vi "Configure.vi"(8 "error in (no error)":errorcluster, 11 "Piezo in":refnum<class "Piezo.lvclass">) -> (0 "error out":errorcluster, 2 "cancelled?":bool, 3 "Piezo out":refnum<class "Piezo.lvclass">)   [LabVIEW 2012, in "Piezo.lvclass"]
doc: "The configure method configures the details for the RabbitMQ connection, the observers and the mapping script.\n\nIn the derived class, make a call to the parent for setting these parameters."
uses:
  Piezo.lvclass
  <vilib>/Utility/miscctls.llb/LVPointTypeDef.ctl
  Piezo.lvclass/Piezo.ctl
  <vilib>/Distrio/Murmex/Murmex/Murmex.lvclass
panel:
  in  "button:call parent":bool
  in  "button:ok":bool
  in  "button:cancel":bool
  in  "Tab Control":enum32{"Task"}(tab)
  in  "Min position":dbl[unit]
  in  "Max position":dbl[unit]
  in  "Reporting folder":path
  in  "Micron to voltage\nconversion factor":dbl[unit]
  in  "Min V":dbl
  in  "Max V":dbl
  in  "Analog output":tag
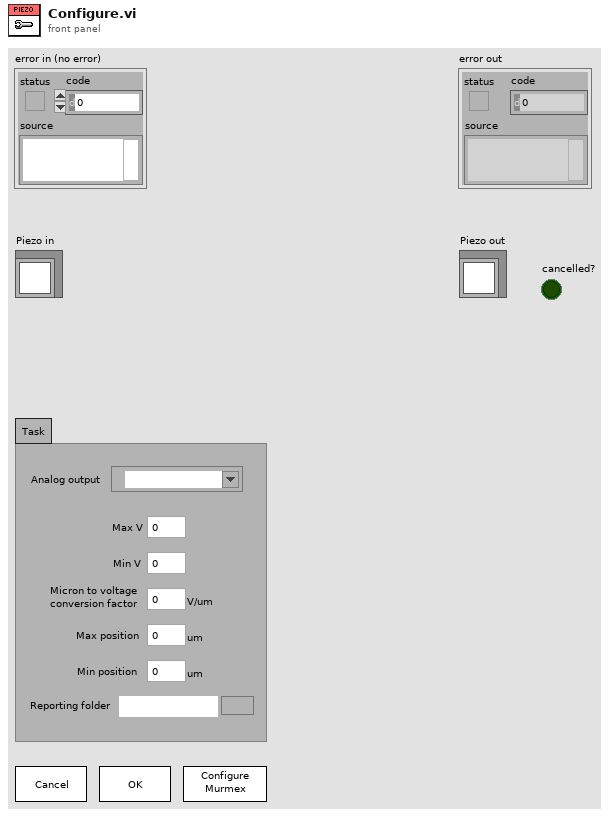
[diagram p1: front panel]
types:
  T1 = typedef "LVPointTypeDef.ctl" = cluster{"Horizontal":i16, "Vertical":i16}
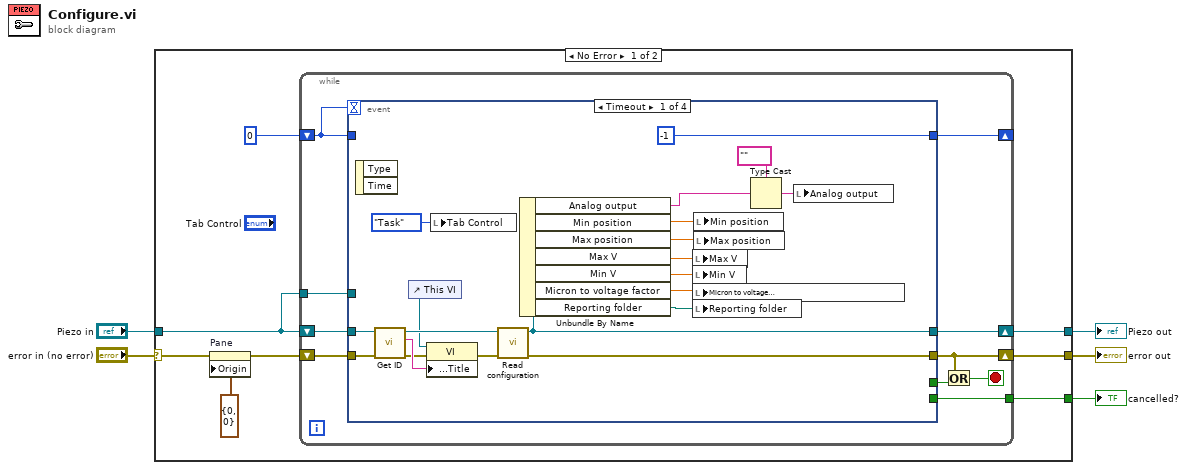
[diagram p0: block diagram]
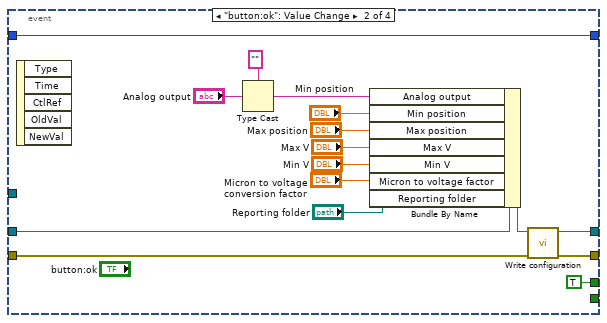
[diagram p2: hidden frame]
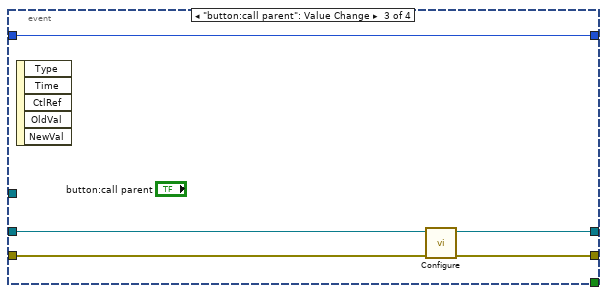
[diagram p3: hidden frame]
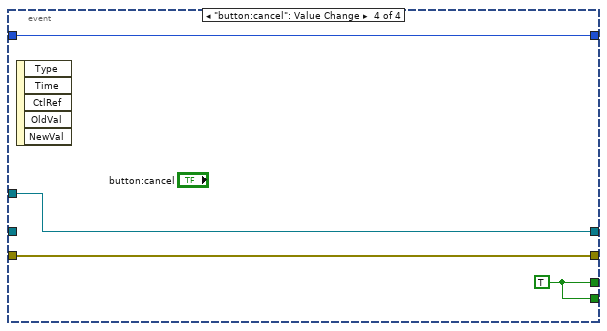
[diagram p4: hidden frame]
diagram:
  n1 = case shown="No Error" "error in (no error)" {
    selector: "error in (no error)" -> [w12 w70]
    tunnel: "Piezo in" -> [w10 w69]
    tunnel: [w7 w70] -> w3
    tunnel: [w8 w69] -> w2
    tunnel: [w6 _] -> w1
    frame No Error {
      n2 = property on="Pane" class="Pane"(error in=w12, "Origin"=T1 {"Horizontal"=0, "Vertical"=0}) -> (error out=w11:errorcluster)  [unwired: 1 in, 1 out]
      n3 = while {
        shift-right: [w17] -> w7
        shift-left: w11 -> [w21]
        shift-right: [w19] -> w8
        shift-left: w10 -> [w20]
        tunnel: w10 -> [w18]
        shift-right: [w22] -> _
        shift-left: 0 -> [w23]
        tunnel: [w14] -> w6
        stop <- w16 stop-if-true
        n4 = event shown="[0] Timeout" {
          selector: _ -> [_ _ _ _]
          dyn-events: _ -> [_ _ _ _]
          timeout: w23 -> [_ _ _ _]
          tunnel: w23 -> [_ w49 w60 w66]
          tunnel: [-1 w49 w60 w66] -> w22
          tunnel: w21 -> [w36 w57 w64 w67]
          tunnel: [w35 w59 w63 w67] -> w17
          tunnel: w20 -> [w34 w56 w61 _]
          tunnel: [w33 w58 w62 w68] -> w19
          tunnel: w18 -> [_ _ _ w68]
          tunnel: [_ TRUE _ w65] -> w15
          tunnel: [_ _ _ w65] -> w14
          event Timeout {
            n5 = event-data() -> ()  [unwired: 1 in, 2 out]
            n6 = call <vilib>:"Get ID.vi"("error in (no error)"=w36, "Murmex in"=w34) -> ("error out"=w37:errorcluster, "component id"=w41:string, "Murmex out"=w40:refnum<class "Piezo.lvclass">)  [unwired: 7 in]
            n7 = control-ref of="This VI"() -> (w38:refnum<vi>)
            n8 = property class="VI"(reference=w38, error in=w37, "Front Panel.Title"=w41) -> (error out=w39:errorcluster)  [unwired: 1 out]
            n9 = local write "Tab Control"(enum32{"Task"}."Task" ("Tab Control")) -> ()
            n10 = call <vilib>:"Read configuration.vi"("error in (no error)"=w39, "Murmex in"=w40) -> ("error out"=w35:errorcluster, "Murmex out"=w33:refnum<class "Piezo.lvclass">)  [unwired: 7 in, 1 out]
            n11 = Unbundle By Name(w33) -> ("Analog output"=w29:string, "Min position"=w25:dbl[unit], "Max position"=w24:dbl[unit], "Max V"=w32:dbl, "Min V"=w31:dbl, "Micron to voltage factor"=w30:dbl[unit], "Reporting folder"=w26:path)
            n12 = local write "Max V"(w32) -> ()
            n13 = local write "Min V"(w31) -> ()
            n14 = local write "Micron to voltage\nconversion factor"(w30) -> ()
            n15 = local write "Reporting folder"(w26) -> ()
            n16 = local write "Min position"(w25) -> ()
            n17 = local write "Max position"(w24) -> ()
            n18 = Type Cast(type=tag "" ("Analog output"), x=w29) -> (*(type *) &x=w27:tag)
            n19 = local write "Analog output"(w27) -> ()
          }
          event "button:ok": Value Change {
            n20 = event-data() -> ()  [unwired: 1 in, 5 out]
            n21 = Type Cast(type="" ("configuration.Analog output"), x="Analog output") -> (*(type *) &x=w52:string)
            n22 = Bundle By Name(cluster=w56, "Analog output"=w52, "Min position"="Min position", "Max position"="Max position", "Max V"="Max V", "Min V"="Min V", "Micron to voltage factor"="Micron to voltage\nconversion factor", "Reporting folder"="Reporting folder") -> (w55:refnum<class "Piezo.lvclass">)
            n23 = call <vilib>:"Write configuration.vi"("error in (no error)"=w57, "Murmex in"=w55) -> ("error out"=w59:errorcluster, "Murmex out"=w58:refnum<class "Piezo.lvclass">)  [unwired: 8 in]
          }
          event "button:call parent": Value Change {
            n24 = event-data() -> ()  [unwired: 1 in, 5 out]
            n25 = call-parent "Configure.vi"("error in (no error)"=w64, "Murmex in"=w61) -> ("error out"=w63:errorcluster, "Murmex out"=w62:refnum<class "Piezo.lvclass">)  [unwired: 7 in, 1 out]
          }
          event "button:cancel": Value Change {
            w65 = TRUE
            n26 = event-data() -> ()  [unwired: 1 in, 5 out]
          }
        }
        n27 = Or(x=w17, y=w15) -> (x .or. y?=w16:bool)
      }
    }
    frame Error {
    }
  }
  "error out" <- w3
  "Piezo out" <- w2
  "cancelled?" <- w1
